vi "Terminate.vi"(8 "error in (no error)":errorcluster, 10 "Message in":refnum<class "TerminateMessage.lvclass">, 11 "Cascade in":refnum<class "Cascade.lvclass">) -> (0 "error out":errorcluster, 3 "Cascade out":refnum<class "Cascade.lvclass">)   [LabVIEW 2012, in "Cascade.lvclass"]
doc: "This member function is called when the statemachine in the run.vi receives an 'terminate' command. It closes the RabbitMQ connection. \n\nOverride this member function in your derived class to release all previously acquired resources (but don't forget to call the parent method). If your component has subcomponents, they count as resources, and you have to release them by calling their own terminate functions."
uses:
  Cascade.lvclass
  <vilib>/Distrio/Murmex/TerminateMessage/TerminateMessage.lvclass
  Cascade.lvclass/Cascade.ctl
  <vilib>/Distrio/Murmex/Murmex/Murmex.lvclass
panel:
  # "This method is called when the TERMINATE\ntrigger is sent. \n\nOverride this method when your component needs to\nrespond to this trigger. \n\nCall parent for proper implementation"
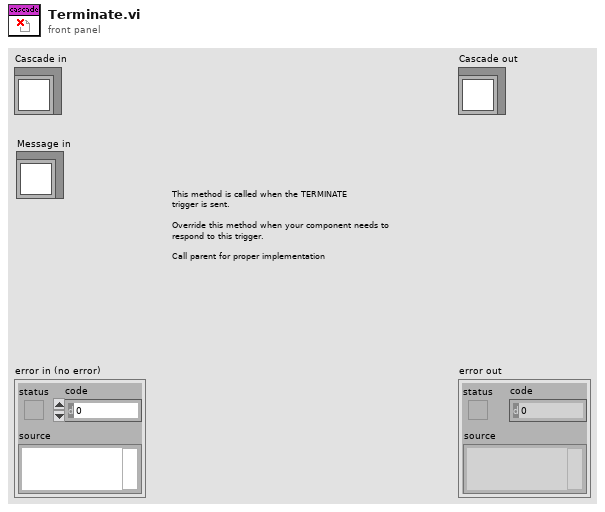
[diagram p1: front panel]
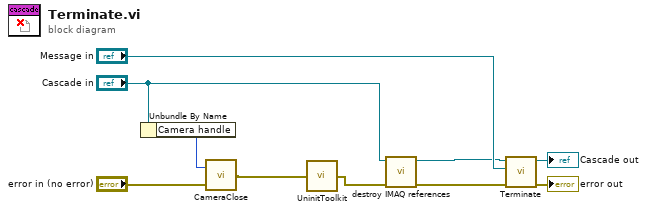
[diagram p0: block diagram]
diagram:
  n1 = Unbundle By Name("Cascade in") -> ("Camera handle"=w6:u32)
  n2 = call <userlib>:"CameraClose.vi"("error in"="error in (no error)", "Camera Handle"=w6) -> ("error out"=w5:errorcluster)
  n3 = call <userlib>:"UninitToolkit.vi"("error in"=w5) -> ("error out"=w3:errorcluster)
  n4 = call-dynamic "destroy IMAQ references.vi"("error in (no error)"=w3, "Cascade in"="Cascade in") -> ("error out"=w4:errorcluster, "Cascade out"=w1:refnum<class "Cascade.lvclass">)  [unwired: 8 in]
  n5 = call-parent "Terminate.vi"("error in (no error)"=w4, "Message in"="Message in", "Murmex in"=w1) -> ("error out"=→"error out":errorcluster, "Murmex out"=→"Cascade out":refnum<class "Cascade.lvclass">)  [unwired: 7 in]
